vi "GetKeyHandle.vi"(8 "error in (no error)":errorcluster, 11 "axis in":cluster{"keyHandle":u32, "nodeId":u16}={"keyHandle"=0, "nodeId"=1}) -> (0 "error out":errorcluster, 3 "keyHandle out":u32)   [LabVIEW 2010]
doc: "<B>GetKeyHandle</B> returns the key handle value."
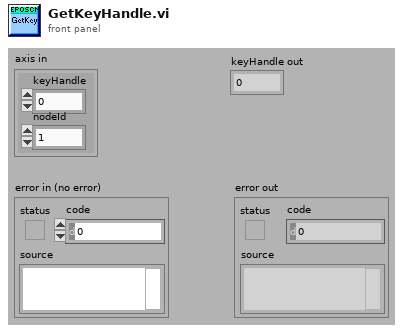
[diagram p1: front panel]
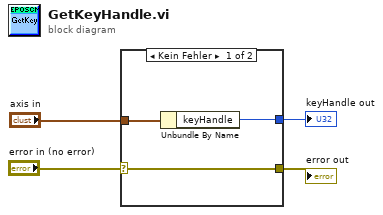
[diagram p0: block diagram]
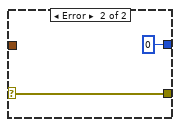
[diagram p2: hidden frame]
diagram:
  n1 = case shown="Kein Fehler" "error in (no error)" {
    selector: "error in (no error)" -> [w5 w9]
    tunnel: [w5 w9] -> w1
    tunnel: "axis in" -> [w7 _]
    tunnel: [w6 u32 0 ("keyHandle")] -> w3
    frame No Error {
      n2 = Unbundle By Name(w7) -> ("keyHandle"=w6:u32)
    }
    frame Error {
    }
  }
  "keyHandle out" <- w3
  "error out" <- w1
